vi "Tosca-Read Parameters.vi"(0 "Path in":path, 11 "error in (no error)":errorcluster, 13 "Prompt? (F)":bool) -> (4 "Path out":path, 6 "Tosca":refnum<class "Parameters.lvclass">, 8 "FSM.Graph":refnum<class "FSM.Graph.lvclass">, 10 "Loaded?":bool, 15 "error out":errorcluster)   [LabVIEW 2020]
uses:
  Classes/Parameters/Parameters.lvclass
  FSM Graph VIs/LV Source/Classes/FSM.Graph/FSM.Graph.lvclass
panel:
  in  "Metadata":cluster{"Version":i32}
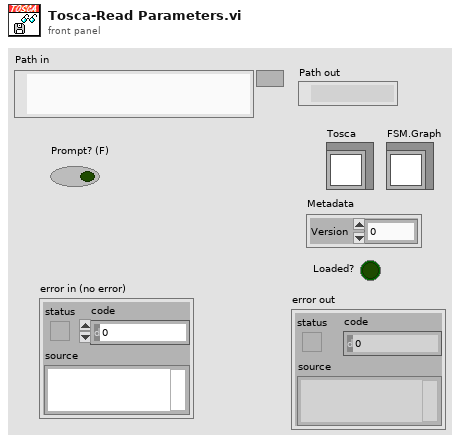
[diagram p1: front panel]
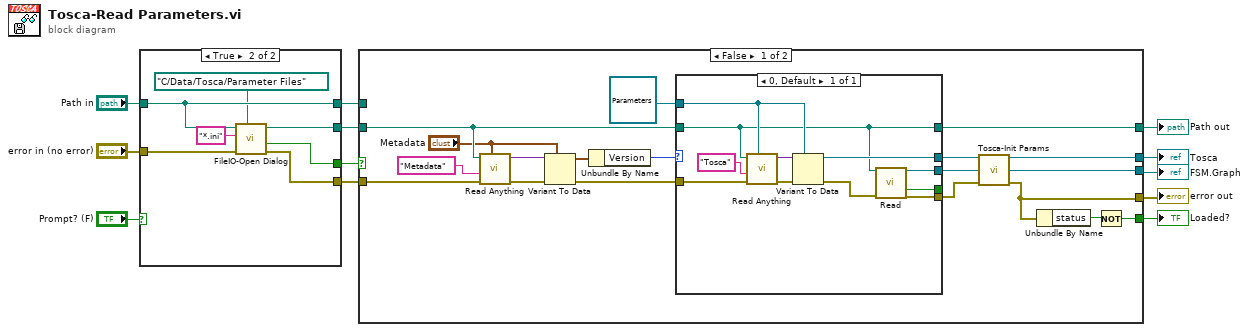
[diagram p0: block diagram]
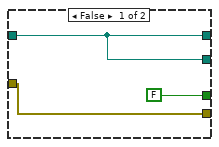
[diagram p2: hidden frame]
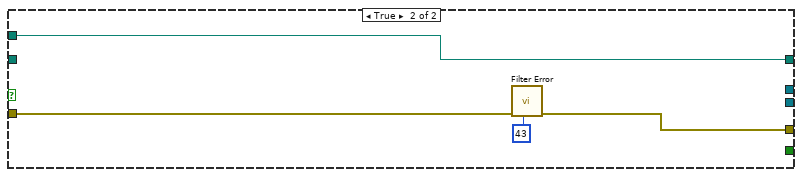
[diagram p3: hidden frame]
diagram:
  n1 = case shown="True" "Prompt? (F)" {
    tunnel: "error in (no error)" -> [w13 w22]
    tunnel: [FALSE ("cancelled") w20] -> w10
    tunnel: [w13 w19] -> w9
    tunnel: [w15 w18] -> w8
    tunnel: "Path in" -> [w15 w17]
    tunnel: [w15 w17] -> w4
    frame False {
    }
    frame True {
      n2 = call "FileIO-Open Dialog.vi"("Default Folder"=path "C:/Data/Tosca/Parameter Files", "error in"=w22, "pattern (all files)"="*.ini", "Start path"=w17) -> ("error out"=w19:errorcluster, "cancelled"=w20:bool, "selected path"=w18:path)  [unwired: 5 in]
    }
  }
  n3 = case shown="False" w10 {
    tunnel: [w25 w53] -> w12
    tunnel: w9 -> [w41 w54]
    tunnel: w8 -> [w38 _]
    tunnel: [w30 w56] -> w6
    tunnel: w4 -> [_ w56]
    tunnel: [w31 _] -> w3
    tunnel: [w27 _] -> w2
    tunnel: [w23 _] -> w1
    frame False {
      n4 = call "Read Anything.vi"("Type of Anything"="Metadata", "Error In"=w41, "Section Name (Name of \"Type of Anything\")"="Metadata" ("Section Name (Name of \"Anything\")"), "Path (dialog)"=w38) -> ("Error Out"=w39:errorcluster, "Anything"=w36:variant)  [unwired: 5 in, 1 out]
      n5 = Variant To Data(error in=w39, type="Metadata", Variant=w36) -> (data=w34:cluster{"Version":i32}, error out=w35:errorcluster)
      n6 = Unbundle By Name(w34) -> ("Version"=w33:i32)
      n7 = case shown="0, Default" w33 {
        tunnel: [w45] -> w26
        tunnel: [w47] -> w28
        tunnel: w38 -> [w44]
        tunnel: w35 -> [w49]
        tunnel: [w44] -> w30
        tunnel: refnum<class "Parameters.lvclass"> refnum ("Tosca") -> [w48]
        tunnel: [w43] -> _
        tunnel: [w42] -> w24
        frame 0, Default {
          n8 = call "Read Anything.vi"("Type of Anything"=w48, "Error In"=w49, "Section Name (Name of \"Type of Anything\")"="Tosca" ("Section Name (Name of \"Anything\")"), "Path (dialog)"=w44) -> ("Error Out"=w51:errorcluster, "Anything"=w50:variant)  [unwired: 5 in, 1 out]
          n9 = Variant To Data(error in=w51, type=w48, Variant=w50) -> (data=w47:refnum<class "Parameters.lvclass">, error out=w46:errorcluster)
          n10 = call "Read.vi"("Path"=w44, "error in (no error)"=w46) -> ("FSM.Graph"=w42:refnum<class "FSM.Graph.lvclass">, "Success"=w43:bool, "error out"=w45:errorcluster)  [unwired: 11 in]
        }
      }
      n11 = call "Tosca-Init Params.vi"("Tosca"=w28, "FSM.Graph"=w24, "error in (no error)"=w26) -> ("Tosca Out"=w27:refnum<class "Parameters.lvclass">, "FSM.Graph Out"=w23:refnum<class "FSM.Graph.lvclass">, "error out"=w25:errorcluster)  [unwired: 10 in]
      n12 = Unbundle By Name(w25) -> ("status"=w32:bool)
      n13 = Not(x=w32) -> (.not. x?=w31:bool)
    }
    frame True {
      n14 = call "Filter Error.vi"("error in (no error)"=w54, "code to ignore"=43) -> ("error out"=w53:errorcluster)  [unwired: 9 in]
    }
  }
  "error out" <- w12
  "Path out" <- w6
  "Loaded?" <- w3
  "Tosca" <- w2
  "FSM.Graph" <- w1
